vi "Create.vi"   [LabVIEW 2021, in "Field_RnD_Services_LIBSSH2_Toolkit.lvlib" / "Known Host.lvclass"]
doc: "Creates a new Known Host object that represents a libssh2lv shared library Known Host struct. This VI must be called, or executed, before using any other Known Host-related VIs. This VI allocates memory within the libssh2lv shared library that must be explicitly deallocated, or freed, at the end of the application using the <B>Destroy</B> VI to avoid memory leaks or running Out-of-Memory (OOM) on a resource contrained system.\n\nA Known Host object represents the read-only data obtained about an entry in a known hosts file on the local host."
uses:
  220524-VNA RP FLAT.llb/Known Host.lvclass
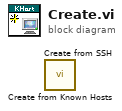
[diagram p0: block diagram]
diagram:
  n1 = call "Create from Known Hosts.vi"() -> ()  [unwired: 9 in, 3 out]
  n2 = call "Create from SSH.vi"() -> ()  [unwired: 10 in, 2 out]
